vi "01-HelloWorld.vi"() -> ()   [LabVIEW 2019]
panel:
  in  "Boolean 2":bool
  out "Boolean":bool
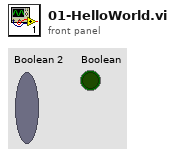
[diagram p1: front panel]
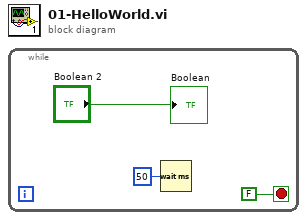
[diagram p0: block diagram]
diagram:
  n1 = while {
    stop <- FALSE stop-if-true
    n2 = Wait (ms)(milliseconds to wait=u32 50) -> ()  [unwired: 1 out]
    "Boolean" <- "Boolean 2"
  }
